vi "Create New GUID.vi"(10 "Error In":errorcluster) -> (2 "Error Out":errorcluster, 3 "New GUID":string)   [LabVIEW 2015, in "Configuration Tool.lvlib"]
doc: "Returns a new GUID"
uses:
  Configuration Tool.lvlib
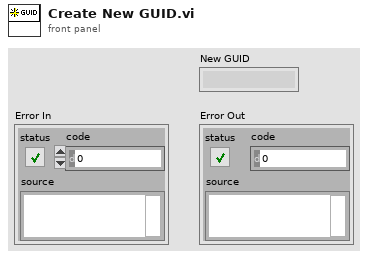
[diagram p1: front panel]
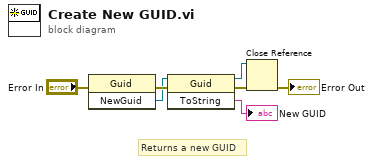
[diagram p0: block diagram]
diagram:
  # "Returns a new GUID"
  n1 = invoke class="Guid" method="NewGuid"(error in="Error In") -> (error out=w4:errorcluster, "NewGuid"=w2:refnum<k24>)  [unwired: 2 in, 1 out]
  n2 = invoke class="Guid" method="ToString"(reference=w2, error in=w4) -> (reference out=w1:refnum<k24>, error out=w5:errorcluster, "ToString"=→"New GUID":string)  [unwired: 1 in]
  n3 = Close Reference(reference=w1, error in (no error)=w5) -> (error out=→"Error Out":errorcluster)
